vi "1553 Address Handles to Write Info.vi"(8 "error in":errorcluster, 11 "Address Based Execution Unit Implementation in":refnum<class "Tx Acyclic Execution Unit.lvclass">) -> (0 "error out":errorcluster, 3 "Address Based Execution Unit Implementation out":refnum<class "Tx Acyclic Execution Unit.lvclass">)   [LabVIEW 2020, in "AIM MIL-STD-1553 Engine.lvlib" / "Implementation.lvlib" / "Tx Acyclic Execution Unit.lvclass"]
uses:
  Tx Acyclic Execution Unit.lvclass
  C:/dev/git/niveristand-aim-milStd1553-custom-device/Source/Custom Device Support/Engine/Implementation/Execution Unit/Execution Unit.lvclass
  Address Write Info.ctl
  Shared/Address.ctl
  Acyclic Trigger Info.ctl
  Execution Unit/Execution Unit.lvclass/Execution Unit.ctl
  Tx Acyclic Execution Unit.lvclass/Tx Acyclic Execution Unit.ctl
  Execution Unit/Execution Unit.lvclass
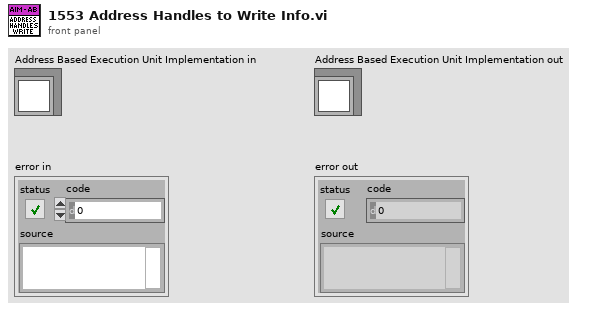
[diagram p1: front panel]
types:
  T1 = typedef "AIM MIL-STD-1553 Engine.lvlib/Implementation.lvlib/Tx Acyclic Execution Unit.lvclass/Acyclic Trigger Info.ctl" = cluster{"bus controller handle":u64, "name":string}
  T2 = typedef "AIM MIL-STD-1553 Engine.lvlib/Implementation.lvlib/Tx Acyclic Execution Unit.lvclass/Address Write Info.ctl" = cluster{"terminal address":T3, "terminal handle":u64}
  T3 = typedef "Address.ctl" = u16
  T4 = typedef "AIM MIL-STD-1553 Engine.lvlib/Implementation.lvlib/Address Based Execution Unit.lvclass/1553 Address Based Handles.ctl" = cluster{"start stop handles":T5[], "acyclic frame trigger handles":T7[]}
  T5 = typedef "AIM MIL-STD-1553 Engine.lvlib/Implementation.lvlib/Address Based Execution Unit.lvclass/Start Stop Channel Handles.ctl" = cluster{"terminal address":T3, "start handle":T6, "stop handle":T6}
  T6 = typedef "Custom Device API.lvlib/Custom Device Item Ref.ctl" = u64
  T7 = typedef "AIM MIL-STD-1553 Engine.lvlib/Implementation.lvlib/Address Based Execution Unit.lvclass/Acyclic Frame Trigger Handle.ctl" = cluster{"name":string, "handle":T6}
  T8 = typedef "AIM MIL-STD-1553 Hardware API.lvlib/Module Reference.ctl" = u32
  T9 = typedef "BIU Configuration.ctl" = cluster{"HW channel":u16, "terminal addresses":T3[], "terminal names":string[], "acyclic frame names":string[], "major frames":T10[], "minor frames":T11[], "messages":T12[]}
  T10 = typedef "Major Frame Definition.ctl" = cluster{"name":string, "minor frames":string[]}
  T11 = typedef "Minor Frame Definition.ctl" = cluster{"name":string, "messages":string[]}
  T12 = typedef "Message Definition.ctl" = cluster{"name":string, "message type":T13, "endpoint Tx":T14, "endpoint Rx":T14, "create timestamp channel":bool, "mode code":u16, "number of words":u16, "parameters":cluster{"name":string, "default value":dbl, "unit":string, "parameter definition":T15}[]}
  T13 = typedef "Message Type.ctl" = string
  T14 = typedef "Terminal Endpoint.ctl" = cluster{"terminal address":T3, "subaddress":T3}
  T15 = typedef "Parameter Definition.ctl" = cluster{"start index":i32, "size (bits)":i32, "encoding":enum16{"BNR", "BCD", "Discrete"}, "signed":bool, "multiplier":dbl, "offset":dbl}
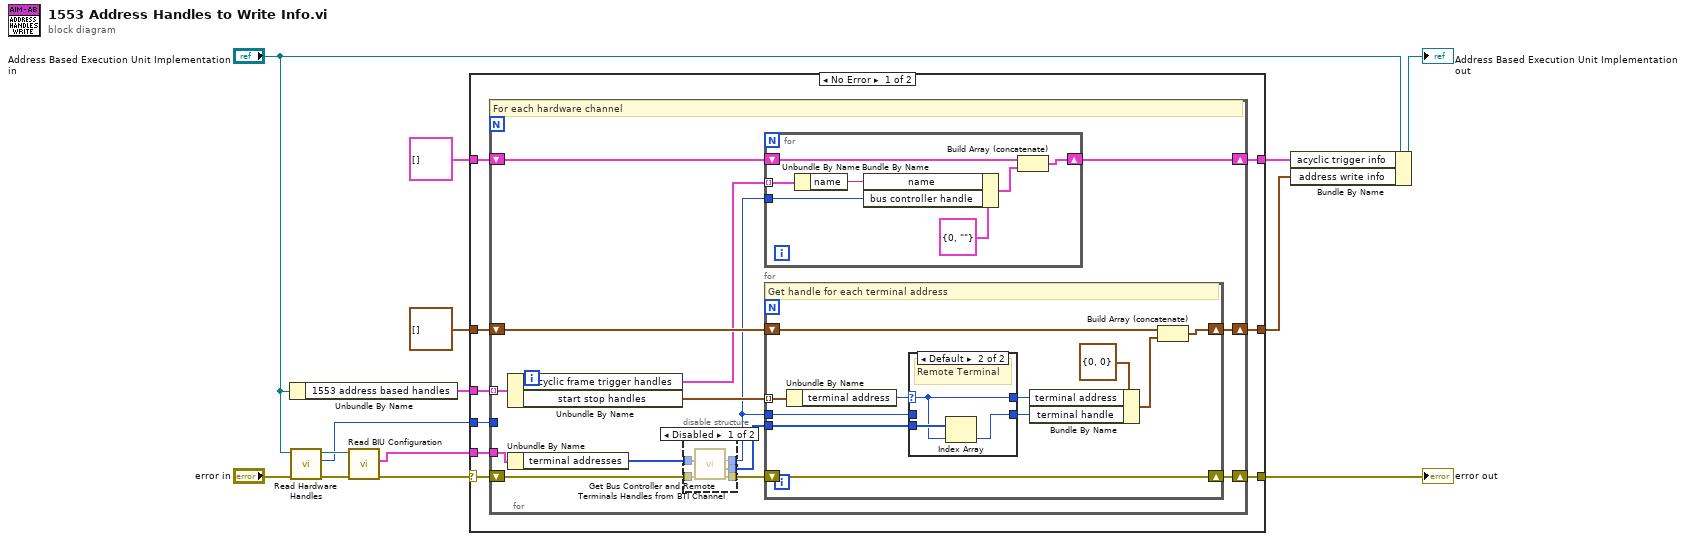
[diagram p0: block diagram]
diagram:
  n1 = Unbundle By Name("Address Based Execution Unit Implementation in") -> ("1553 address based handles"=w6:T4[])
  n2 = call "Read Hardware Handles.vi"("error in"="error in", "Execution Unit in"="Address Based Execution Unit Implementation in") -> ("error out"=w10:errorcluster, "module reference"=w7:T8, "Execution Unit out"=w8:refnum<class "Tx Acyclic Execution Unit.lvclass">)  [unwired: 7 in]
  n3 = call "Read BIU Configuration.vi"("error in"=w10, "execution unit"=w8) -> ("error out"=w11:errorcluster, "biu configuration"=w12:T9)  [unwired: 7 in, 1 out]
  n4 = case shown="No Error" w11 {
    selector: w11 -> [w22 w67]
    tunnel: w12 -> [w19 _]
    tunnel: w7 -> [w23 _]
    tunnel: [w21 w67] -> w14
    tunnel: w6 -> [w20 _]
    tunnel: T2[] [] ("address write info") -> [w18 _]
    tunnel: [w17 _] -> w3
    tunnel: T1[] [] -> [w16 _]
    tunnel: [w15 _] -> w1
    frame No Error {
      n5 = for {
        tunnel: w19 -> [w37]
        tunnel: w23 -> [_]
        shift-right: [w36] -> w21
        shift-left: w22 -> [w29]
        tunnel: w20 -> [w32] mode=indexing
        shift-right: [w33] -> w17
        shift-left: w18 -> [w34]
        shift-right: [w30] -> w15
        shift-left: w16 -> [w31]
        # "For each hardware channel"
        n6 = Unbundle By Name(w32) -> ("acyclic frame trigger handles"=w25:T7[], "start stop handles"=w35:T5[])
        n7 = Unbundle By Name(w37) -> ("terminal addresses"=w24:T3[])
        n8 = disable-structure shown="Disabled" {
          disable-tunnel: w29 -> [w42 w43]
          disable-tunnel: [w41 w43] -> w28
          disable-tunnel: [w40 _] -> w27
          disable-tunnel: [w39 _] -> w26
          disable-tunnel: w24 -> [w38 _]
          frame Disabled {
            n9 = call "Get Bus Controller and Remote Terminals Handles from BTI Channel.vi"("error in"=w42, "terminal addresses"=w38) -> ("error out"=w41:errorcluster, "remote terminal handles out"=w40:u64[], "bus controller handle out"=w39:u64)  [unwired: 6 in, 1 out]
          }
          frame Enabled {
          }
        }
        n10 = for {
          tunnel: w25 -> [w50] mode=indexing
          tunnel: w26 -> [w47]
          shift-right: [w45] -> w30
          shift-left: w31 -> [w48]
          n11 = Unbundle By Name(w50) -> ("name"=w44:string)
          n12 = Bundle By Name(cluster=T1 {"bus controller handle"=0, "name"=""} ("acyclic trigger info"), "name"=w44, "bus controller handle"=w47) -> (w46:T1)
          n13 = Build Array (concatenate)(w48, w46) -> (w45:T1[])
        }
        n14 = for {
          shift-right: [w61] -> w36
          shift-left: w28 -> [w61]
          tunnel: w27 -> [w59]
          tunnel: w35 -> [w60] mode=indexing
          tunnel: w26 -> [w57]
          shift-right: [w51] -> w33
          shift-left: w34 -> [w53]
          # "Get handle for each terminal address"
          n15 = Unbundle By Name(w60) -> ("terminal address"=w58:T3)
          n16 = case shown="Default" w58 {
            selector: w58 -> [w62 w64]
            tunnel: w59 -> [_ w66]
            tunnel: [w63 w65] -> w54
            tunnel: w57 -> [w63 _]
            tunnel: [w62 w64] -> w55
            frame 0 {
              # "Bus Controller"
            }
            frame Default {
              # "Remote Terminal"
              n17 = Index Array(array=w66, index=w64) -> (element=w65:u64)
            }
          }
          n18 = Bundle By Name(cluster=T2 {"terminal address"=0, "terminal handle"=0} ("address write info"), "terminal address"=w55, "terminal handle"=w54) -> (w52:T2)
          n19 = Build Array (concatenate)(w53, w52) -> (w51:T2[])
        }
      }
    }
    frame Error {
    }
  }
  "error out" <- w14
  n20 = Bundle By Name(cluster="Address Based Execution Unit Implementation in", "acyclic trigger info"=w1, "address write info"=w3) -> (→"Address Based Execution Unit Implementation out":refnum<class "Tx Acyclic Execution Unit.lvclass">)
